vi "CRYAna 2ch ScanFFT.vi"(8 "EQ information":T2={"Stimulus EQ Curve"={"Name"="", "Curve"=[], "X data"=1, "Y data"=1, "Z data"=1, "X axis"=0, "Y axis"=1, "Z axis"=1, "X unit"="Hz", "Y unit"="", "Z unit"="deg.", "X dB ref"=1.0, "Y dB ref"=1.0, "Z dB ref"=1.0, "single val"=FALSE, "protected"=FALSE, "display X"=TRUE, "display Y"=TRUE, "display Z"=TRUE, "Test Info"="", "Step No."=0, "Plot Settings"={"Color"=0, "Interpolation"=0, "Point Style"=0, "Line Style"=0, "Point Color"=0, "Line Width"=0, "Bar Plot Style"=0, "Fill To"=0}, "AutoProtect"=FALSE}, "EQ"=FALSE, "EQ Rate"=0.0} {"EQ Rate" format="%.2f"; "Stimulus EQ Curve"."Z data" items=["dB", "Lin"]; "Stimulus EQ Curve"."X data" items=["dB", "Lin"]; "Stimulus EQ Curve"."Y data" items=["dB", "Lin"]; "Stimulus EQ Curve"."Z dB ref" format="%.1f"; "Stimulus EQ Curve"."Z axis" items=["Log", "Lin"]; "Stimulus EQ Curve"."X dB ref" format="%.1f"; "Stimulus EQ Curve"."X axis" items=["Log", "Lin"]; "Stimulus EQ Curve"."Y axis" items=["Log", "Lin"]; "Stimulus EQ Curve"."Y dB ref" format="%.1f"; "Stimulus EQ Curve"."Curve"."z" format="%.2f"; "Stimulus EQ Curve"."Curve"."y" format="%.2f"; "Stimulus EQ Curve"."Curve"."x" format="%.2f"}, 9 "In Parameter":T3={"Fs(Hz)"=44100.0, "dF(Hz)"=5.0, "Overlap(%)"=75.0, "Window"=1} {"Window" items=["Rectangle"=0, "Hanning"=1, "Hamming"=2, "Blackman-Harris"=3, "Exact Blackman"=4, "Blackman"=5, "Flat Top"=6, "4 Term B-Harris "=7, "7 Term B-Harris"=8, "Low Sidelobe"=9, "Blackman Nuttall"=11, "Triangle"=30, "Bartlett-Hanning"=31, "Bohman"=32, "Parzen"=33, "Welch"=34, "Kaiser"=60, "Dolph-Chebyshev"=61, "Gaussian"=62]}, 10 "Response[y(t)]":dbl[](array[numeric]) format="%.2f", 11 "Stimulus[x(t)]":dbl[](array[numeric]) format="%.2f") -> (0 "New dF(Hz)":dbl=44100.0, 1 "Gyy":dbl[](array[numeric]) format="%#_6p", 2 "Gxy":cdb[](array[numeric]) format="%#_1p", 3 "Gxx":dbl[](array[numeric]) format="%#_3p")   [LabVIEW 2013]
uses:
  Typedef Control/CRYData Cluster.ctl
  <vilib>/Analysis/2dsp.llb/Real FFT.vi
  <vilib>/Analysis/0measdsp.llb/Scaled Time Domain Window (DBL).vi
  <vilib>/Analysis/NI_AALPro.lvlib
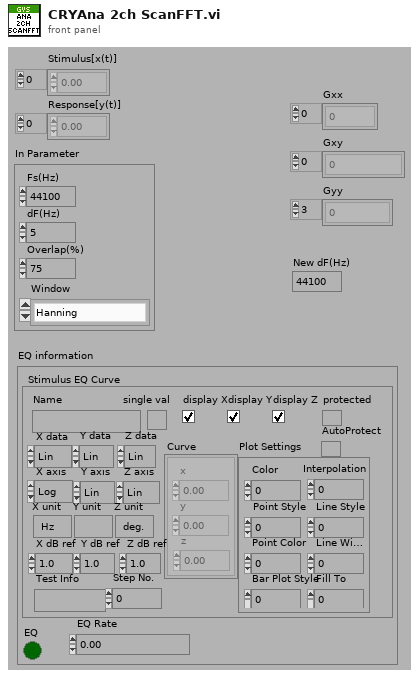
[diagram p1: front panel]
types:
  T1 = typedef "CRYData Cluster.ctl" = cluster{"Name":string, "Curve":cluster{"x":dbl, "y":dbl, "z":dbl}[], "X data":u16, "Y data":u16, "Z data":u16, "X axis":u16, "Y axis":u16, "Z axis":u16, "X unit":string, "Y unit":string, "Z unit":string, "X dB ref":dbl, "Y dB ref":dbl, "Z dB ref":dbl, "single val":bool, "protected":bool, "display X":bool, "display Y":bool, "display Z":bool, "Test Info":string, "Step No.":i32, "Plot Settings":cluster{"Color":u32, "Interpolation":u8, "Point Style":u8, "Line Style":u8, "Point Color":u32, "Line Width":u8, "Bar Plot Style":u8, "Fill To":i16}, "AutoProtect":bool}
  T2 = cluster{"Stimulus EQ Curve":T1, "EQ":bool, "EQ Rate":dbl}
  T3 = cluster{"Fs(Hz)":dbl, "dF(Hz)":dbl, "Overlap(%)":dbl, "Window":u32}
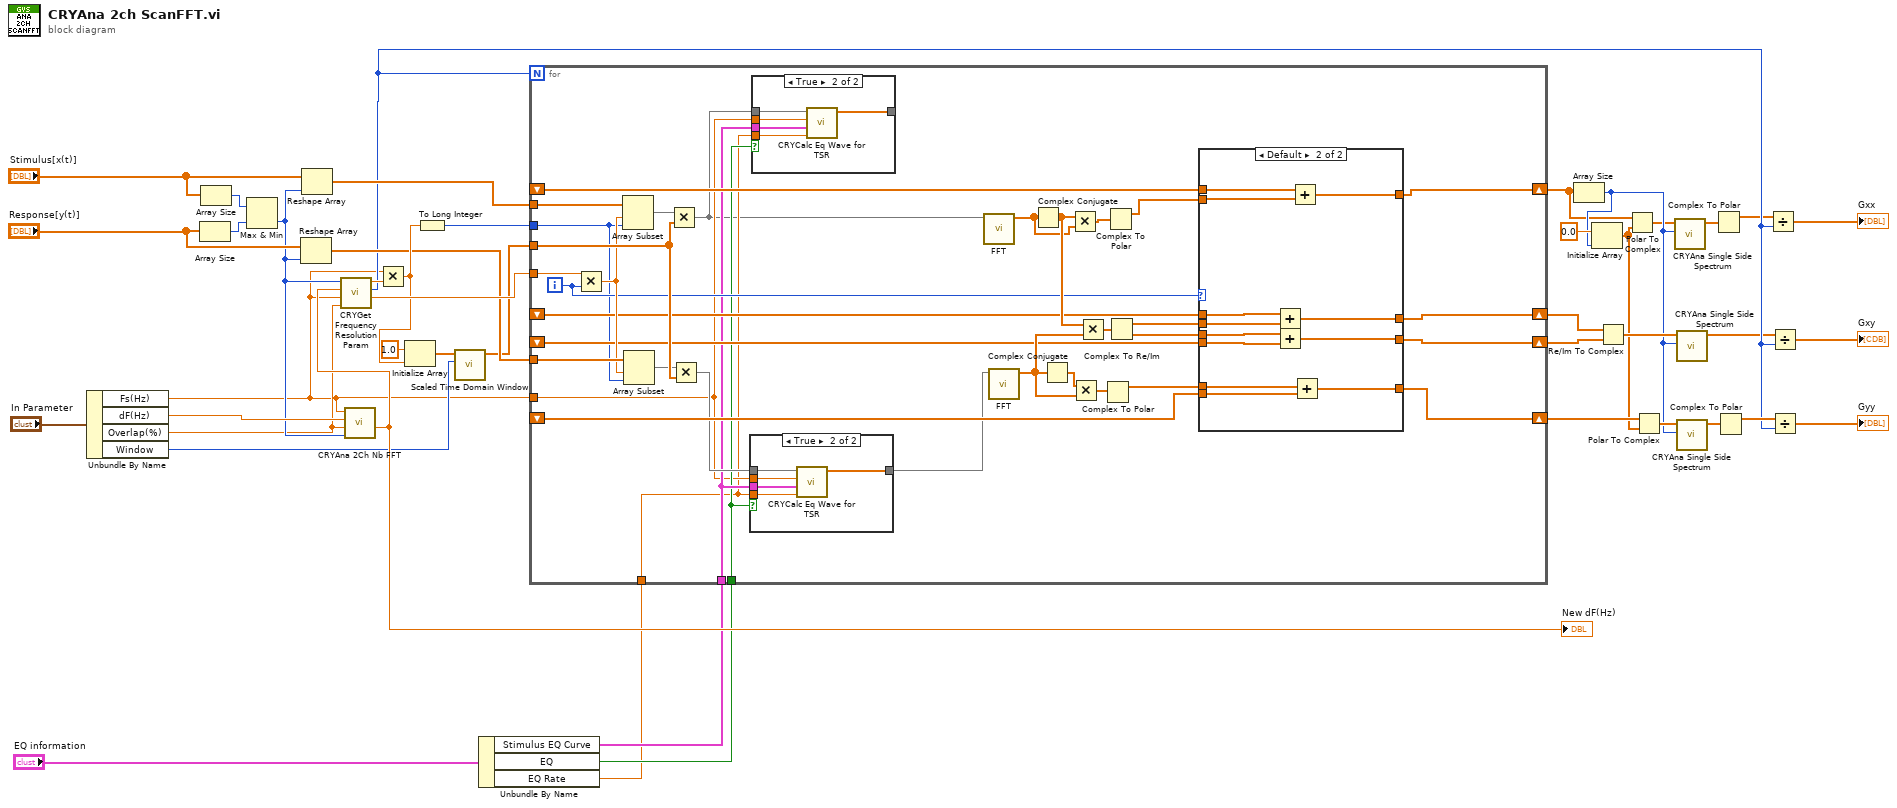
[diagram p0: block diagram]
diagram:
  n1 = Unbundle By Name("In Parameter") -> ("Fs(Hz)"=w2:dbl, "dF(Hz)"=w43:dbl, "Overlap(%)"=w9:dbl, "Window"=w8:u32)
  n2 = Array Size(array="Response[y(t)]") -> (size(s)=w42:i32)
  n3 = Array Size(array="Stimulus[x(t)]") -> (size(s)=w41:i32)
  n4 = Max & Min(x=w41, y=w42) -> (min(x,y)=w11:i32)  [unwired: 1 out]
  n5 = Reshape Array("Response[y(t)]", w11) -> (w34:dbl[])
  n6 = Reshape Array("Stimulus[x(t)]", w11) -> (w35:dbl[])
  n7 = call "CRYAna 2Ch Nb FFT.vi"("Wave Size (Sp)"=w11, "Overlap (%)"=w9, "dF(Hz)"=w43, "Fs(Hz)"=w2) -> ("New dF (Hz)"=w10:dbl)  [unwired: 4 in, 3 out]
  "New dF(Hz)" <- w10
  n8 = call "CRYGet Frequency Resolution Param.vi"("Overlap(%)"=w9, "Fs"=w2, "Freq Resolution(Hz)"=w10, "Samples"=w11) -> ("Shift Samples"=w39:dbl, "No. of FFT"=w16:i32, "Record Length(s)"=w40:dbl)  [unwired: 4 in, 1 out]
  n9 = Multiply(x=w2, y=w40) -> (x*y=w36:dbl)
  n10 = Initialize Array(1.0 ("element"), w36) -> (w37:dbl[])
  n11 = To Long Integer(number=w36) -> (32bit integer=w24:i32)
  n12 = call-poly <vilib>:"Scaled Time Domain Window.vi"("window"=w8, "X"=w37) -> ("Windowed X"=w27:dbl[])  [unwired: 7 in, 2 out]
  n13 = Unbundle By Name("EQ information") -> ("Stimulus EQ Curve"=w4:T1, "EQ"=w3:bool, "EQ Rate"=w1:dbl)
  n14 = for {
    N: w16 -> [_]
    tunnel: w35 -> [w76]
    tunnel: w39 -> [w74]
    tunnel: w24 -> [w53]
    shift-right: [w78] -> w18
    shift-left: _ -> [w77]
    tunnel: w27 -> [w73]
    shift-right: [w62] -> w32
    shift-left: _ -> [w63]
    tunnel: w34 -> [w75]
    shift-right: [w59] -> w29
    shift-left: _ -> [w61]
    shift-right: [w58] -> w33
    shift-left: _ -> [w56]
    tunnel: w4 -> [w48]
    tunnel: w3 -> [w47]
    tunnel: w1 -> [w45]
    tunnel: w2 -> [w46]
    i -> [w54]
    n15 = Multiply(x=w74, y=w54) -> (x*y=w72:dbl)
    n16 = Array Subset(array=w76, index=w72, length=w53) -> (w52:dbl[])
    n17 = Array Subset(array=w75, index=w72, length=w53) -> (w51:dbl[])
    n18 = Multiply(x=w52, y=w73) -> (x*y=w44:dbl[])
    n19 = Multiply(x=w51, y=w73) -> (x*y=w50:dbl[])
    n20 = case shown="True" w47 {
      tunnel: w48 -> [_ w90]
      tunnel: w46 -> [_ w89]
      tunnel: w45 -> [_ w88]
      tunnel: w50 -> [w85 w87]
      tunnel: [w85 w86] -> w49
      frame False {
      }
      frame True {
        n21 = call "CRYCalc Eq Wave for TSR.vi"("EQ Rate"=w88, "EQ Curve"=w90, "Fs"=w89, "Wave In"=w87) -> ("Wave Out"=w86:dbl[])  [unwired: 6 in, 1 out]
      }
    }
    n22 = case shown="True" w47 {
      tunnel: w48 -> [_ w84]
      tunnel: w46 -> [_ w83]
      tunnel: w45 -> [_ w82]
      tunnel: w44 -> [w79 w81]
      tunnel: [w79 w80] -> _
      frame False {
      }
      frame True {
        n23 = call "CRYCalc Eq Wave for TSR.vi"("EQ Rate"=w82, "EQ Curve"=w84, "Fs"=w83, "Wave In"=w81) -> ("Wave Out"=w80:dbl[])  [unwired: 6 in, 1 out]
      }
    }
    n24 = call-poly <vilib>:"FFT.vi"("X"=w44) -> ("FFT {X}"=w66:cdb[])  [unwired: 2 in, 8 out]
    n25 = call-poly <vilib>:"FFT.vi"("X"=w49) -> ("FFT {X}"=w65:cdb[])  [unwired: 2 in, 8 out]
    n26 = Complex Conjugate(1:w66) -> (0:w67:cdb[])
    n27 = Complex Conjugate(1:w65) -> (0:w69:cdb[])
    n28 = Multiply(x=w67, y=w66) -> (x*y=w70:cdb[])
    n29 = Multiply(x=w69, y=w65) -> (x*y=w68:cdb[])
    n30 = Multiply(x=w67, y=w65) -> (x*y=w64:cdb[])
    n31 = Complex To Polar(r * e^(i*theta)=w68) -> (r=w55:dbl[])  [unwired: 1 out]
    n32 = Complex To Polar(r * e^(i*theta)=w70) -> (r=w71:dbl[])  [unwired: 1 out]
    n33 = Complex To Re/Im(x + iy=w64) -> (x=w60:dbl[], y=w57:dbl[])
    n34 = case shown="Default" w54 {
      tunnel: w71 -> [w94 w104]
      tunnel: [w94 w105] -> w78
      tunnel: w77 -> [_ w106]
      tunnel: w55 -> [w93 w103]
      tunnel: w63 -> [_ w102]
      tunnel: [w93 w101] -> w62
      tunnel: w61 -> [_ w100]
      tunnel: w60 -> [w92 w99]
      tunnel: [w92 w98] -> w59
      tunnel: [w91 w97] -> w58
      tunnel: w57 -> [w91 w96]
      tunnel: w56 -> [_ w95]
      frame 0 {
      }
      frame Default {
        n35 = Add(x=w100, y=w99) -> (x+y=w98:dbl[])
        n36 = Add(x=w96, y=w95) -> (x+y=w97:dbl[])
        n37 = Add(x=w106, y=w104) -> (x+y=w105:dbl[])
        n38 = Add(x=w103, y=w102) -> (x+y=w101:dbl[])
      }
    }
  }
  n39 = Array Size(array=w18) -> (size(s)=w19:i32)
  n40 = Initialize Array(0.0 ("element"), w19) -> (w17:dbl[])
  n41 = Re/Im To Complex(1:w33, 2:w29) -> (0:w28:cdb[])
  n42 = Polar To Complex(1:w17, 2:w18) -> (0:w6:cdb[])
  n43 = Polar To Complex(1:w17, 2:w32) -> (0:w31:cdb[])
  n44 = call "CRYAna Single Side Spectrum.vi"("FFT Size"=w19, "FFT"=w6) -> ("Single FFT"=w26:cdb[])  [unwired: 8 in, 1 out]
  n45 = call "CRYAna Single Side Spectrum.vi"("FFT Size"=w19, "FFT"=w28) -> ("Single FFT"=w15:cdb[])  [unwired: 8 in, 1 out]
  n46 = call "CRYAna Single Side Spectrum.vi"("FFT Size"=w19, "FFT"=w31) -> ("Single FFT"=w25:cdb[])  [unwired: 8 in, 1 out]
  n47 = Complex To Polar(r * e^(i*theta)=w26) -> (r=w7:dbl[])  [unwired: 1 out]
  n48 = Complex To Polar(r * e^(i*theta)=w25) -> (r=w22:dbl[])  [unwired: 1 out]
  n49 = Divide(x=w7, y=w16) -> (x/y=→"Gxx":dbl[])
  n50 = Divide(x=w15, y=w16) -> (x/y=→"Gxy":cdb[])
  n51 = Divide(x=w22, y=w16) -> (x/y=→"Gyy":dbl[])
